vi "InitActor.vi"() -> (5 "Actor":refnum<class "Actor.lvclass">)   [LabVIEW 2020, in "jettl.lvlib" / "Base.lvlib"]
uses:
  Base.lvlib
  Actor/Actor.lvclass
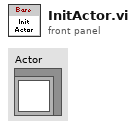
[diagram p1: front panel]
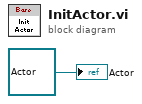
[diagram p0: block diagram]
diagram:
  "Actor" <- refnum<class "Actor.lvclass"> refnum ("jettl.lvlib:Base.lvlib:Actor.lvclass")
